vi "Send Record Trace.vi"(7 "Message Priority (Normal)":T1=enum."Normal", 8 "error in (no error)":errorcluster, 10 "Trace":refnum<class "Trace.lvclass">, 11 "Message Enqueuer":refnum<class "Message Enqueuer.lvclass">) -> (0 "error out":errorcluster, 3 "Message Enqueuer out":refnum<class "Message Enqueuer.lvclass">)   [LabVIEW 2014, in "Robot Actor Framework.lvlib" / "System Actor.lvlib" / "Record Trace Msg.lvclass"]
doc: "This VI sends the message to an actor."
uses:
  Record Trace Msg.lvclass
  <vilib>/ActorFramework/Message Enqueuer/Message Enqueuer.lvclass
  <vilib>/ActorFramework/Message Enqueuer/Message Priority.ctl
  Trace/Trace Class/Trace.lvclass
  Record Trace Msg.lvclass/Record Trace Msg.ctl
  <vilib>/ActorFramework/Message Enqueuer/Message Enqueuer.lvclass/Message Enqueuer.ctl
  <vilib>/ActorFramework/Message Priority Queue/Priority Enqueue.vi
  Utilities/Utilities.lvlib
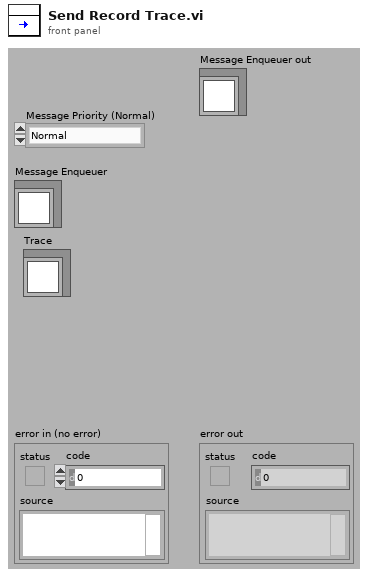
[diagram p1: front panel]
types:
  T1 = typedef "Actor Framework.lvlib/Message Enqueuer.lvclass/Message Priority.ctl" = enum16{"Low", "Normal", "High"}
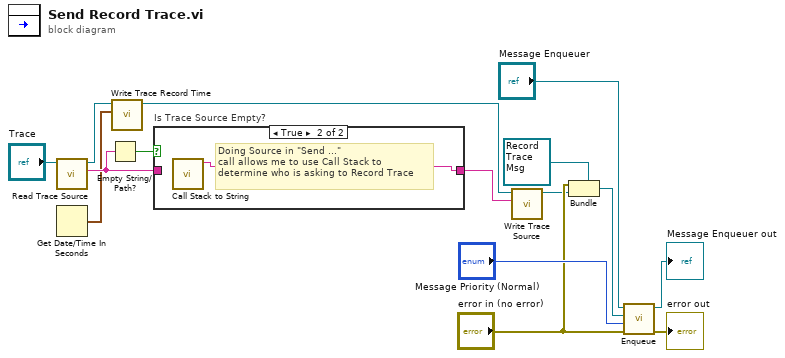
[diagram p0: block diagram]
diagram:
  n1 = call-dynamic "Read Trace Source.vi"("Trace in"="Trace") -> ("Trace Source"=w5:string, "Trace out"=w4:refnum<class "Trace.lvclass">)  [unwired: 8 in, 1 out]
  n2 = Get Date/Time In Seconds() -> (seconds since 1Jan1904=w2:timestamp)
  n3 = Empty String/Path?(string/path=w5) -> (empty?=w9:bool)
  n4 = call-dynamic "Write Trace Record Time.vi"("Trace Record Time"=w2, "Trace in"=w4) -> ("Trace out"=w3:refnum<class "Trace.lvclass">)  [unwired: 8 in, 1 out]
  n5 = case "Is Trace Source Empty?" shown="True" w9 {
    tunnel: [w16 w17] -> w8
    tunnel: w5 -> [w16 _]
    frame False {
    }
    frame True {
      # "Doing Source in \"Send ...\"\ncall allows me to use Call Stack to \ndetermine who is asking to Record Trace"
      n6 = call "Call Stack to String.vi"() -> ("Call Stack String"=w17:string)  [unwired: 11 in]
    }
  }
  n7 = call-dynamic "Write Trace Source.vi"("Trace Source"=w8, "Trace in"=w3) -> ("Trace out"=w1:refnum<class "Trace.lvclass">)  [unwired: 8 in, 1 out]
  n8 = Bundle(cluster=refnum<class "Record Trace Msg.lvclass"> refnum ("Object"), "error in (no error)", w1) -> (w12:refnum<class "Record Trace Msg.lvclass">)
  n9 = call <vilib>:"Enqueue.vi"("error in (no error)"="error in (no error)", "Message Priority (Normal)"="Message Priority (Normal)", "Message"=w12, "Message Enqueuer in"="Message Enqueuer") -> ("error out"=→"error out":errorcluster, "Message Enqueuer out"=→"Message Enqueuer out":refnum<class "Message Enqueuer.lvclass">)  [unwired: 6 in]
